vi "LVLIBRev.vi"() -> (4 "Path":string="C:\\Test Engr\\Instrument Drivers\\Vitrek V7X\\LVLIBRev.vi", 8 "Version":string="2.0.0.0")   [LabVIEW 2010, in "VITREK V7X.lvlib"]
uses:
  VITREK V7X.lvlib
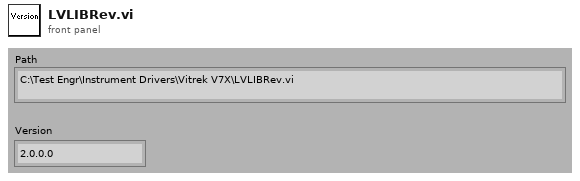
[diagram p1: front panel]
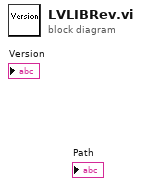
[diagram p0: block diagram]
diagram:
